vi "Open Library.vi"(8 "error in (no error)":errorcluster, 10 "Full Path":path, 11 "Application in":refnum<vi>) -> (0 "error out":errorcluster, 2 "Library out":refnum<vi>, 3 "Application out":refnum<vi>)   [LabVIEW 2019, in "VI Scripting Tools.lvlib"]
uses:
  VI Scripting Tools.lvlib
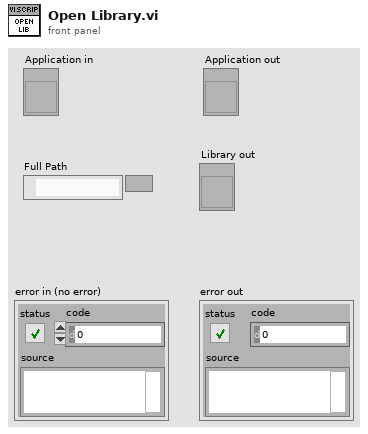
[diagram p1: front panel]
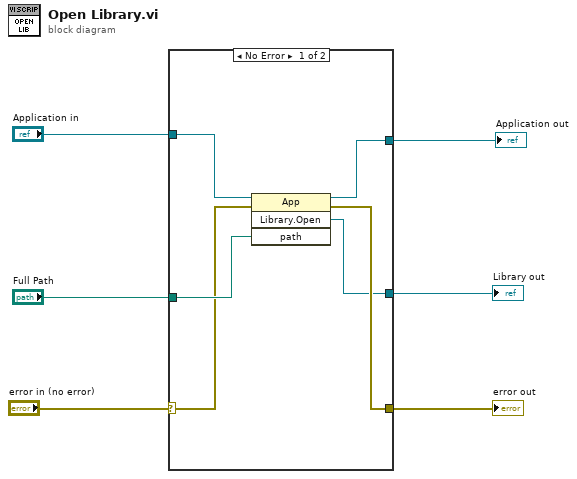
[diagram p0: block diagram]
diagram:
  n1 = case shown="No Error" "error in (no error)" {
    selector: "error in (no error)" -> [w7 w13]
    tunnel: [w12 w13] -> w6
    tunnel: "Full Path" -> [w11 _]
    tunnel: "Application in" -> [w10 w14]
    tunnel: [w9 _] -> w3
    tunnel: [w8 w14] -> w2
    frame No Error {
      n2 = invoke class="App" method="Library.Open"(reference=w10, error in=w7, "path"=w11) -> (reference out=w8:refnum<vi>, error out=w12:errorcluster, "Open Library"=w9:refnum<vi>)  [unwired: 1 in, 1 out]
    }
    frame Error {
    }
  }
  "error out" <- w6
  "Library out" <- w3
  "Application out" <- w2
